vi "Timeout.vi"(8 "error in (no error)":errorcluster, 11 "Active in":refnum<class "Active.lvclass">) -> (0 "error out":errorcluster, 3 "State Actor out":refnum<class "State Actor.lvclass">)   [LabVIEW 2024, in "Sample State Actor.lvlib" / "Active.lvclass"]
uses:
  Active.lvclass
  State Actor/State Actor.lvclass
  Timed Out/Timed Out.lvclass
  C:/Users/ottoa/OneDrive/Desktop/working copies/stateActor/src/State Actor/State Actor.lvclass
  Active.lvclass/Active.ctl
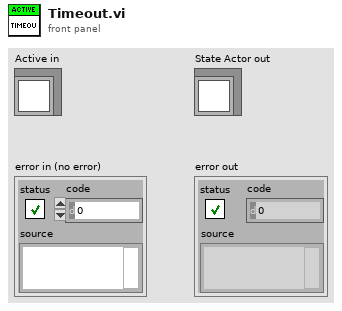
[diagram p1: front panel]
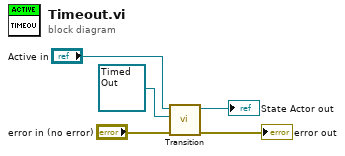
[diagram p0: block diagram]
diagram:
  n1 = call-dynamic "Transition.vi"("error in (no error)"="error in (no error)", "Target State Actor in"=refnum<class "Timed Out.lvclass"> refnum ("Sample State Actor.lvlib:Timed Out.lvclass"), "State Actor in"="Active in") -> ("error out"=→"error out":errorcluster, "State Actor out"=→"State Actor out":refnum<class "State Actor.lvclass">)  [unwired: 7 in]
